vi "Add.vi"(7 "LabVIEW Web Service Request":refnum<class "Web Request.lvclass">, 10 "b":dbl format="%#_13g", 11 "a":dbl format="%#_13g") -> (2 "value":string, 3 "c":dbl)   [LabVIEW 2015]
uses:
  <vilib>/wsapi/Web Request.lvclass
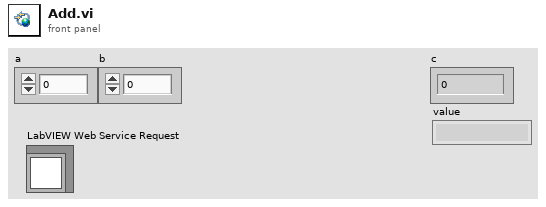
[diagram p1: front panel]
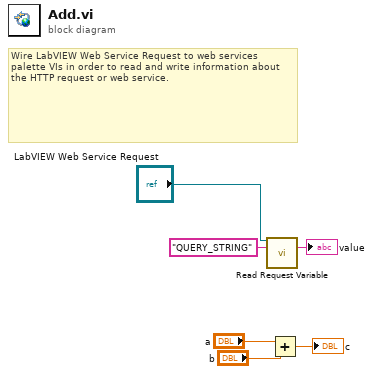
[diagram p0: block diagram]
diagram:
  # "Wire LabVIEW Web Service Request to web services palette VIs in order to read and write information about the HTTP request or web service."
  n1 = call <vilib>:"Read Request Variable.vi"("LabVIEW Web Service Request"="LabVIEW Web Service Request", "variable name"="QUERY_STRING") -> ("value"=→"value":string)  [unwired: 11 in, 2 out]
  n2 = Add(x="a", y="b") -> (x+y=→"c":dbl)
